vi "SRG.vi"(0 "System no.":i32=1 min=1 max=4 step=1, 2 "Axis to set":string[](array[string]), 3 "Register value":dbl[](array[numeric]) format="%.6f", 4 "No.of digits":i16=4, 5 "error in":errorcluster, 6 "Register number":i32[](array[numeric])) -> (14 "Controller error":bool, 19 "error out":errorcluster)   [LabVIEW 2020]
doc: "Sets register values for commanded axes, waits 100 ms and queries ERR?. See system manual for available parameter numbers and values. No. of digits is the number of digits after the decimal point in the register value(s) that will be sent. Controller error is TRUE if selected system reports an error code which is not 0."
panel:
  # "This vi sets register values, waits 100 ms and queries ERR?. See system manual \nfor available register numbers and values."
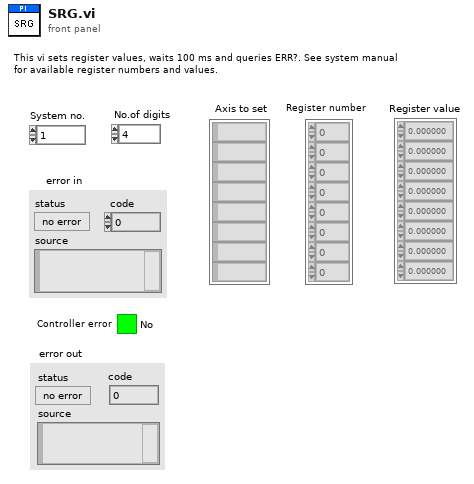
[diagram p1: front panel]
types:
  T1 = enum16{"Disable error check", "Force error check", "Use global settings"}
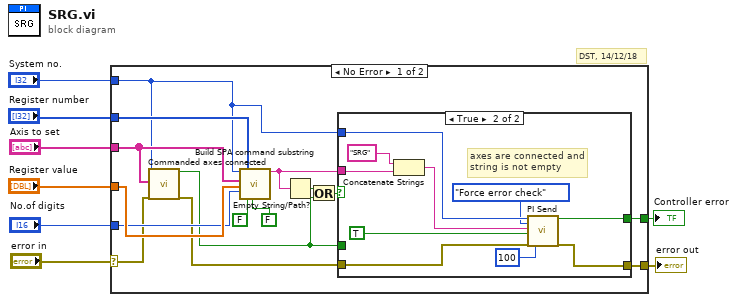
[diagram p0: block diagram]
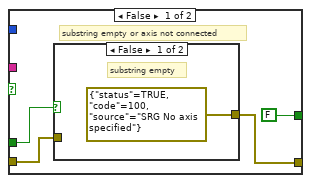
[diagram p2: hidden frame]
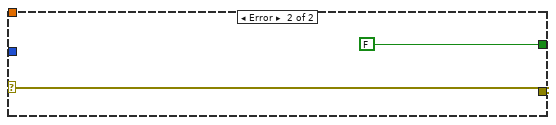
[diagram p4: hidden frame]
diagram:
  # "DST, 14/12/18"
  n1 = case shown="No Error" "error in" {
    selector: "error in" -> [w11 w41]
    tunnel: [w23 w41] -> w8
    tunnel: "Register value" -> [w22 _]
    tunnel: "No.of digits" -> [w21 _]
    tunnel: "System no." -> [w9 _]
    tunnel: "Axis to set" -> [w18 _]
    tunnel: "Register number" -> [w17 _]
    tunnel: [w10 FALSE ("Controller error")] -> w1
    frame No Error {
      n2 = call "Commanded axes connected.vi"("System no."=w9, "Commanded axes"=w18, "error in"=w11) -> ("Controller error"=w14:bool, "error out"=w20:errorcluster)  [unwired: 1 in, 14 out]
      n3 = call "Build SPA command substring.vi"("System no."=w9, "Axes to set"=w18, "Parameter values"=w22, "No. of digits"=w21, "Parameter number"=w17, "Parameter no. format \n(Decimal: FALSE)"=FALSE ("Parameter no. format \n(Decimal: FALSE)"), "Parameter format \n(Num.: FALSE)"=FALSE ("Parameter format \n(Num.: FALSE)")) -> ("SPA command substring"=w13:string)  [unwired: 3 in, 9 out]
      n4 = Empty String/Path?(string/path=w13) -> (empty?=w12:bool)
      n5 = Or(x=w12, y=w14) -> (x .or. y?=w19:bool)
      n6 = case shown="True" w19 {
        tunnel: w13 -> [_ w38]
        tunnel: [w27 w31] -> w23
        tunnel: w20 -> [w25 w35]
        tunnel: w14 -> [w26 _]
        tunnel: w9 -> [_ w34]
        tunnel: [FALSE ("Controller error") w30] -> w10
        frame False {
          # "substring empty or axis not connected"
          n7 = case shown="False" w26 {
            tunnel: [errorcluster {"status"=TRUE, "code"=100, "source"="SRG No axis specified"} ("error out") w29] -> w27
            tunnel: w25 -> [_ w29]
            frame False {
              # "substring empty"
            }
            frame True {
              # "commanded axis not connected"
            }
          }
        }
        frame True {
          # "axes are connected and\nstring is not empty"
          n8 = Concatenate Strings("SRG", w38) -> (w36:string)
          n9 = call "PI Send.vi"("System no."=w34, "Error check settings"=T1."Force error check", "String to send"=w36, "Attach termination char.?"=TRUE ("Attach Linefeed?"), "error in"=w35, "Delay before error check (ms)"=u32 100) -> ("Controller error"=w30:bool, "error out"=w31:errorcluster)  [unwired: 12 out]
        }
      }
    }
    frame Error {
    }
  }
  "error out" <- w8
  "Controller error" <- w1
